vi "test-median-filter.vi"(8 "error in (no error)":errorcluster) -> (0 "error out":errorcluster, 3 "ALL TESTS PASSED":bool)   [LabVIEW 2019]
uses:
  <vilib>/Rock Robotics/WPI/ThirdParty/JAS_Junk/TrajLib/MEDIAN_FILTER.ctl
  <vilib>/Rock Robotics/WPI/ThirdParty/JAS_Junk/TrajLib/Trajectory_Library.lvlib
panel:
  out "Passed 3":bool
  out "Passed 2":bool
  out "Passed 1":bool
  out "Passed 0":bool
  out "MedianValue 6 = 3.5":dbl
  out "MedianValue 5 = 3":dbl
  out "MedianValue 4 = 1.5":dbl
  out "MedianValue  3  = 0":dbl
  out "MedianValue 2 = 1.5":dbl
  out "MedianValue   1 = 3":dbl
  out "Out MEDIAN_FILTER 2":T1 {"ValueBuffer" format="%13.5g"}
  out "T3--X--Value":dbl
  out "T3 -- X -- 0":dbl
  out "Out MEDIAN_FILTER":T1 {"ValueBuffer" format="%13.5g"}
  out "T2--X--Value":dbl
  out "T0--X--Value":dbl
  out "T2 -- X -- 0":dbl
  out "T1 -- X -- 0":dbl
  out "T0 -- X -- 0":dbl
  # "Median Filter Test"
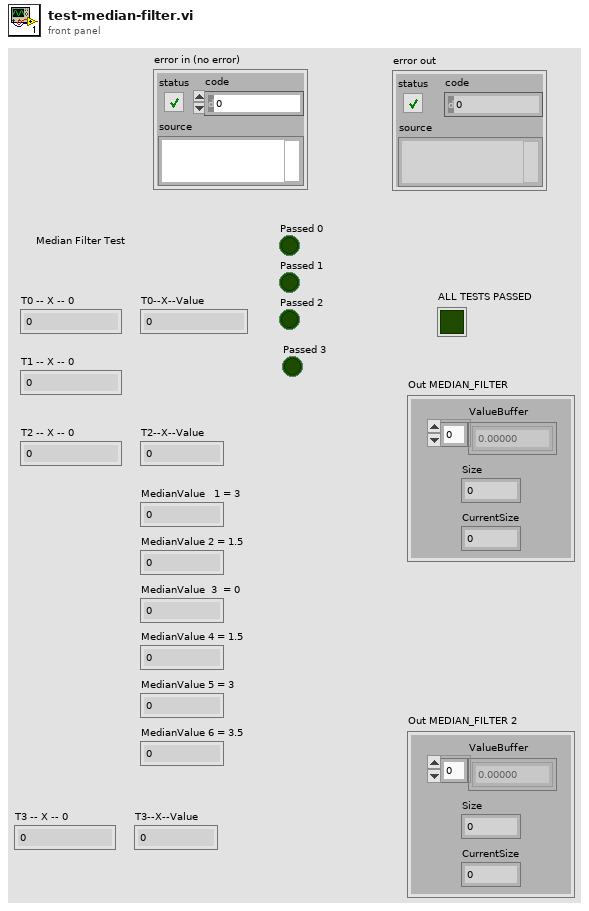
[diagram p1: front panel]
types:
  T1 = typedef "Trajectory_Library.lvlib/MEDIAN_FILTER.ctl" = cluster{"ValueBuffer":dbl[], "Size":i32, "CurrentSize":i32}
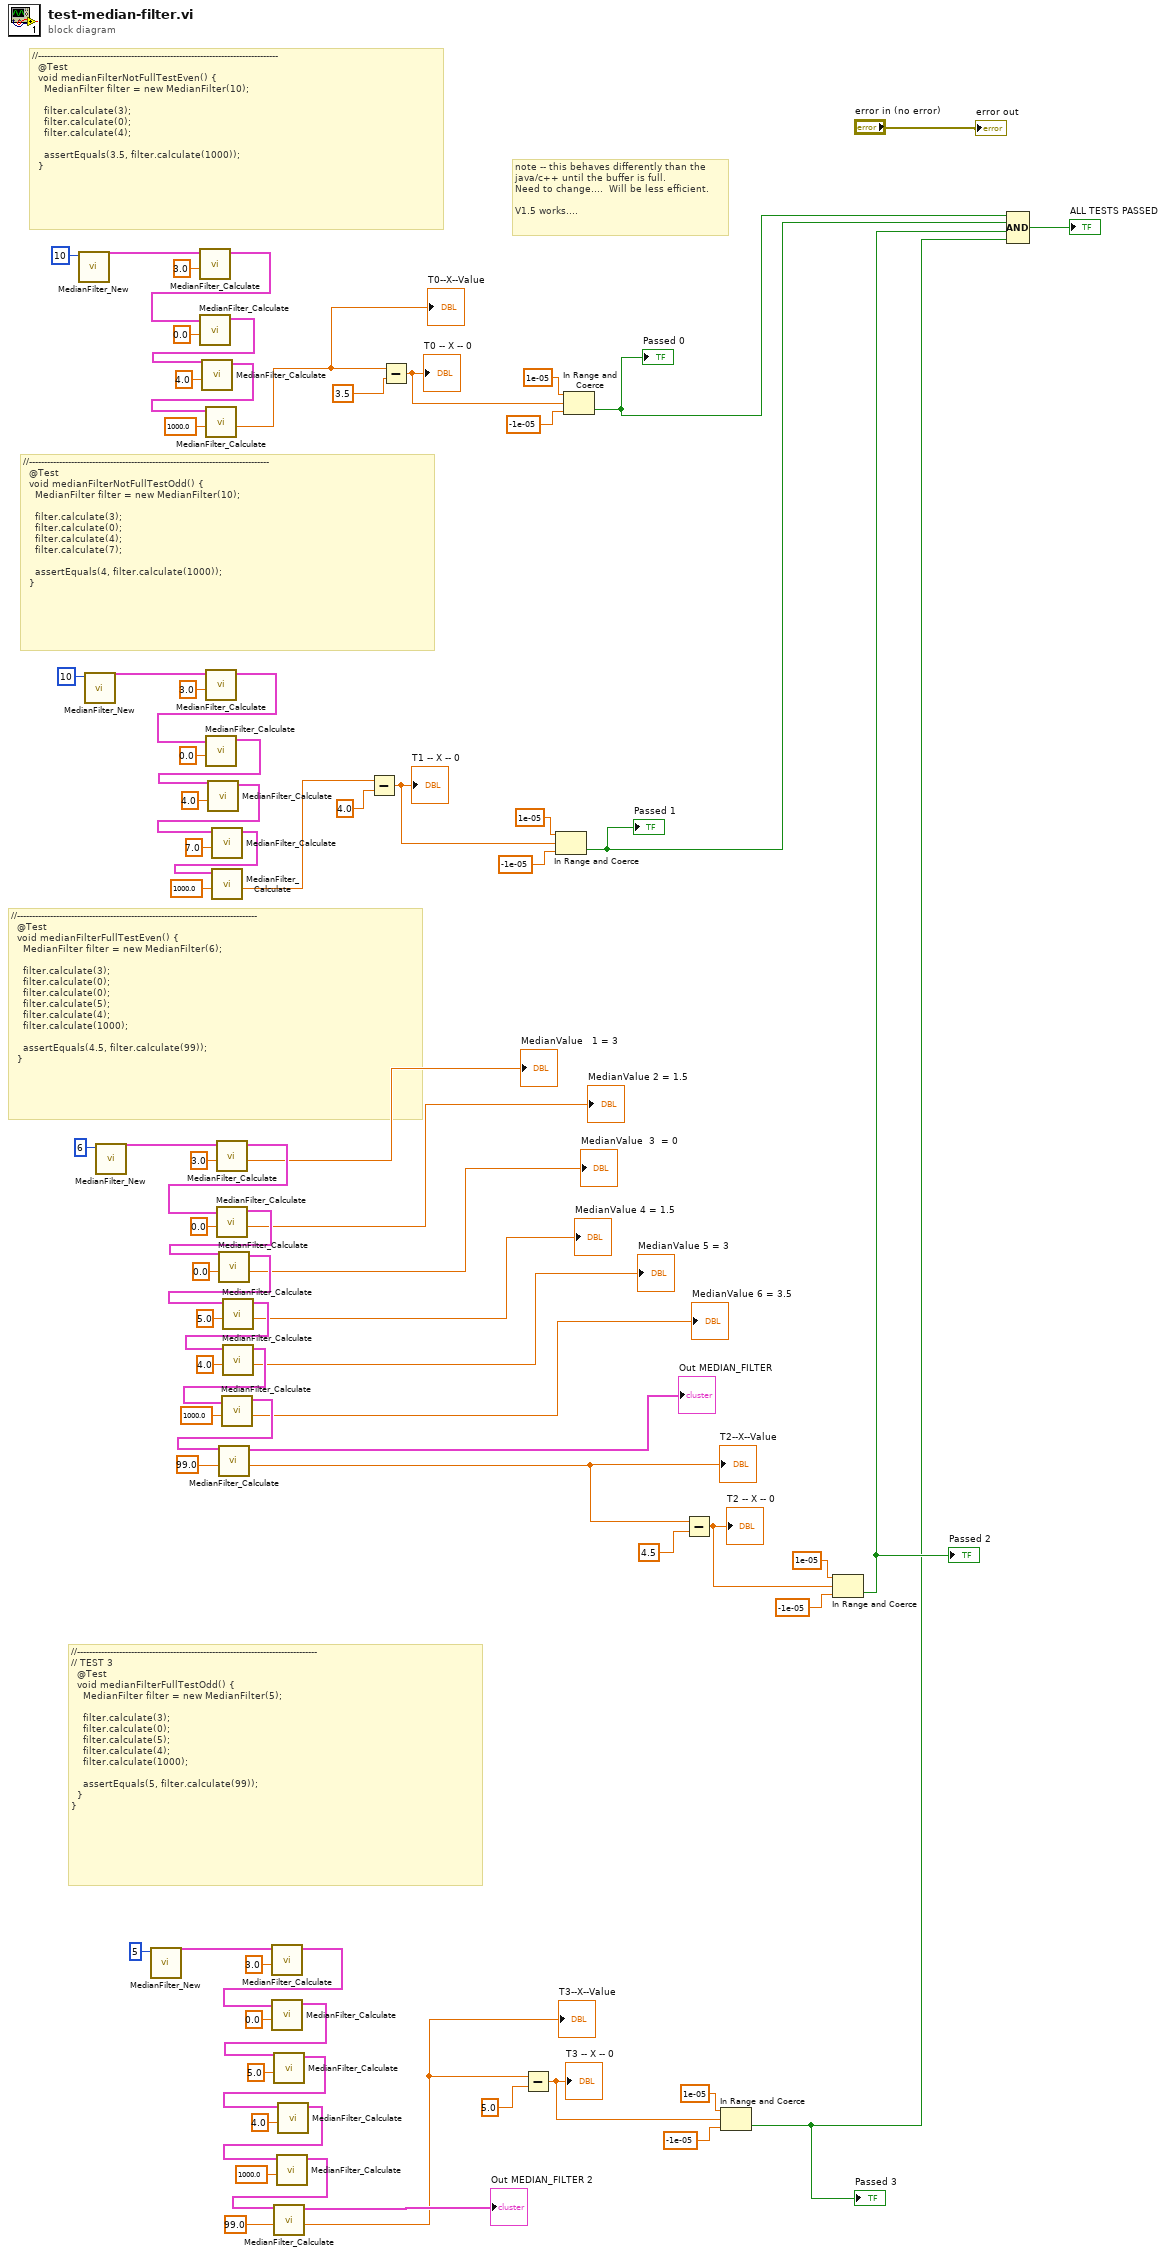
[diagram p0: block diagram]
diagram:
  # "//--------------------------------------------------------------------------------\n// TEST 3\n  @Test\n  void medianFilterFullTestOdd() {\n    MedianFilter filter = new MedianFilter(5);\n\n    filter.calculate(3);\n    filter.calculate(0);\n    filter.calculate(5);\n    filter.calculate(4);\n    filter.calculate(1000);\n\n    assertEquals(5, filter.calculate(99));\n  }\n}"
  # "note -- this behaves differently than the \njava/c++ until the buffer is full.\nNeed to change....  Will be less efficient.\n\nV1.5 works...."
  # "//--------------------------------------------------------------------------------\n  @Test\n  void medianFilterFullTestEven() {\n    MedianFilter filter = new MedianFilter(6);\n\n    filter.calculate(3);\n    filter.calculate(0);\n    filter.calculate(0);\n    filter.calculate(5);\n    filter.calculate(4);\n    filter.calculate(1000);\n\n    assertEquals(4.5, filter.calculate(99));\n  }"
  # "//--------------------------------------------------------------------------------\n  @Test\n  void medianFilterNotFullTestOdd() {\n    MedianFilter filter = new MedianFilter(10);\n\n    filter.calculate(3);\n    filter.calculate(0);\n    filter.calculate(4);\n    filter.calculate(7);\n\n    assertEquals(4, filter.calculate(1000));\n  }"
  # "//--------------------------------------------------------------------------------\n  @Test\n  void medianFilterNotFullTestEven() {\n    MedianFilter filter = new MedianFilter(10);\n\n    filter.calculate(3);\n    filter.calculate(0);\n    filter.calculate(4);\n\n    assertEquals(3.5, filter.calculate(1000));\n  }"
  n1 = call <vilib>:"MedianFilter_New.vi"("Samples"=10) -> ("MEDIAN_FILTER"=w76:T1)  [unwired: 10 in]
  n2 = call <vilib>:"MedianFilter_New.vi"("Samples"=10) -> ("MEDIAN_FILTER"=w67:T1)  [unwired: 10 in]
  n3 = call <vilib>:"MedianFilter_New.vi"("Samples"=6) -> ("MEDIAN_FILTER"=w54:T1)  [unwired: 10 in]
  n4 = call <vilib>:"MedianFilter_New.vi"("Samples"=5) -> ("MEDIAN_FILTER"=w38:T1)  [unwired: 10 in]
  n5 = call <vilib>:"MedianFilter_Calculate.vi"("Input Value"=3.0, "In MEDIAN_FILTER"=w76) -> ("Out MEDIAN_FILTER"=w75:T1)  [unwired: 8 in, 1 out]
  n6 = call <vilib>:"MedianFilter_Calculate.vi"("Input Value"=0.0, "In MEDIAN_FILTER"=w75) -> ("Out MEDIAN_FILTER"=w74:T1)  [unwired: 8 in, 1 out]
  n7 = call <vilib>:"MedianFilter_Calculate.vi"("Input Value"=4.0, "In MEDIAN_FILTER"=w74) -> ("Out MEDIAN_FILTER"=w73:T1)  [unwired: 8 in, 1 out]
  n8 = call <vilib>:"MedianFilter_Calculate.vi"("Input Value"=1000.0, "In MEDIAN_FILTER"=w73) -> ("MedianValue"=w81:dbl)  [unwired: 8 in, 1 out]
  "T0--X--Value" <- w81
  n9 = call <vilib>:"MedianFilter_Calculate.vi"("Input Value"=3.0, "In MEDIAN_FILTER"=w67) -> ("Out MEDIAN_FILTER"=w66:T1)  [unwired: 8 in, 1 out]
  n10 = call <vilib>:"MedianFilter_Calculate.vi"("Input Value"=0.0, "In MEDIAN_FILTER"=w66) -> ("Out MEDIAN_FILTER"=w65:T1)  [unwired: 8 in, 1 out]
  n11 = call <vilib>:"MedianFilter_Calculate.vi"("Input Value"=4.0, "In MEDIAN_FILTER"=w65) -> ("Out MEDIAN_FILTER"=w64:T1)  [unwired: 8 in, 1 out]
  n12 = call <vilib>:"MedianFilter_Calculate.vi"("Input Value"=7.0, "In MEDIAN_FILTER"=w64) -> ("Out MEDIAN_FILTER"=w62:T1)  [unwired: 8 in, 1 out]
  n13 = call <vilib>:"MedianFilter_Calculate.vi"("Input Value"=1000.0, "In MEDIAN_FILTER"=w62) -> ("MedianValue"=w60:dbl)  [unwired: 8 in, 1 out]
  n14 = call <vilib>:"MedianFilter_Calculate.vi"("Input Value"=3.0, "In MEDIAN_FILTER"=w54) -> ("MedianValue"=→"MedianValue   1 = 3":dbl, "Out MEDIAN_FILTER"=w53:T1)  [unwired: 8 in]
  n15 = call <vilib>:"MedianFilter_Calculate.vi"("Input Value"=0.0, "In MEDIAN_FILTER"=w53) -> ("MedianValue"=→"MedianValue 2 = 1.5":dbl, "Out MEDIAN_FILTER"=w52:T1)  [unwired: 8 in]
  n16 = call <vilib>:"MedianFilter_Calculate.vi"("Input Value"=0.0, "In MEDIAN_FILTER"=w52) -> ("MedianValue"=→"MedianValue  3  = 0":dbl, "Out MEDIAN_FILTER"=w51:T1)  [unwired: 8 in]
  n17 = call <vilib>:"MedianFilter_Calculate.vi"("Input Value"=5.0, "In MEDIAN_FILTER"=w51) -> ("MedianValue"=→"MedianValue 4 = 1.5":dbl, "Out MEDIAN_FILTER"=w49:T1)  [unwired: 8 in]
  n18 = call <vilib>:"MedianFilter_Calculate.vi"("Input Value"=4.0, "In MEDIAN_FILTER"=w49) -> ("MedianValue"=→"MedianValue 5 = 3":dbl, "Out MEDIAN_FILTER"=w47:T1)  [unwired: 8 in]
  n19 = call <vilib>:"MedianFilter_Calculate.vi"("Input Value"=1000.0, "In MEDIAN_FILTER"=w47) -> ("MedianValue"=→"MedianValue 6 = 3.5":dbl, "Out MEDIAN_FILTER"=w45:T1)  [unwired: 8 in]
  n20 = call <vilib>:"MedianFilter_Calculate.vi"("Input Value"=99.0, "In MEDIAN_FILTER"=w45) -> ("MedianValue"=w22:dbl, "Out MEDIAN_FILTER"=→"Out MEDIAN_FILTER":T1)  [unwired: 8 in]
  "T2--X--Value" <- w22
  n21 = call <vilib>:"MedianFilter_Calculate.vi"("Input Value"=3.0, "In MEDIAN_FILTER"=w38) -> ("Out MEDIAN_FILTER"=w37:T1)  [unwired: 8 in, 1 out]
  n22 = call <vilib>:"MedianFilter_Calculate.vi"("Input Value"=0.0, "In MEDIAN_FILTER"=w37) -> ("Out MEDIAN_FILTER"=w36:T1)  [unwired: 8 in, 1 out]
  n23 = call <vilib>:"MedianFilter_Calculate.vi"("Input Value"=5.0, "In MEDIAN_FILTER"=w36) -> ("Out MEDIAN_FILTER"=w35:T1)  [unwired: 8 in, 1 out]
  n24 = call <vilib>:"MedianFilter_Calculate.vi"("Input Value"=4.0, "In MEDIAN_FILTER"=w35) -> ("Out MEDIAN_FILTER"=w30:T1)  [unwired: 8 in, 1 out]
  n25 = call <vilib>:"MedianFilter_Calculate.vi"("Input Value"=1000.0, "In MEDIAN_FILTER"=w30) -> ("Out MEDIAN_FILTER"=w32:T1)  [unwired: 8 in, 1 out]
  n26 = call <vilib>:"MedianFilter_Calculate.vi"("Input Value"=99.0, "In MEDIAN_FILTER"=w32) -> ("MedianValue"=w21:dbl, "Out MEDIAN_FILTER"=→"Out MEDIAN_FILTER 2":T1)  [unwired: 8 in]
  "T3--X--Value" <- w21
  n27 = Subtract(x=w60, y=4.0) -> (x-y=w14:dbl)
  "T1 -- X -- 0" <- w14
  n28 = Subtract(x=w81, y=3.5) -> (x-y=w3:dbl)
  "T0 -- X -- 0" <- w3
  n29 = Subtract(x=w21, y=5.0) -> (x-y=w7:dbl)
  "T3 -- X -- 0" <- w7
  n30 = In Range and Coerce(upper limit=1e-05, x=w14, lower limit=-1e-05) -> (In Range?=w5:bool)  [unwired: 1 out]
  "Passed 1" <- w5
  n31 = In Range and Coerce(upper limit=1e-05, x=w3, lower limit=-1e-05) -> (In Range?=w6:bool)  [unwired: 1 out]
  "Passed 0" <- w6
  n32 = Subtract(x=w22, y=4.5) -> (x-y=w10:dbl)
  "T2 -- X -- 0" <- w10
  n33 = In Range and Coerce(upper limit=1e-05, x=w7, lower limit=-1e-05) -> (In Range?=w2:bool)  [unwired: 1 out]
  "Passed 3" <- w2
  n34 = In Range and Coerce(upper limit=1e-05, x=w10, lower limit=-1e-05) -> (In Range?=w4:bool)  [unwired: 1 out]
  "Passed 2" <- w4
  n35 = Compound Arithmetic op=AND(w6, w5, w4, w2) -> (→"ALL TESTS PASSED":bool)
  "error out" <- "error in (no error)"
